vi "Read_spec_No_of_Characters.vi"(0 "Filename":path) -> (1 "character string":string, 2 "Error?":bool)   [LabVIEW 2020]
panel:
  out "error out":errorcluster
  out "Bytes to read":i32
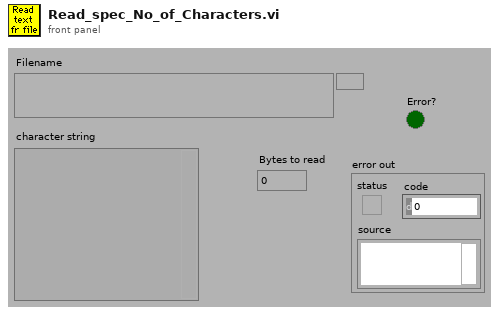
[diagram p1: front panel]
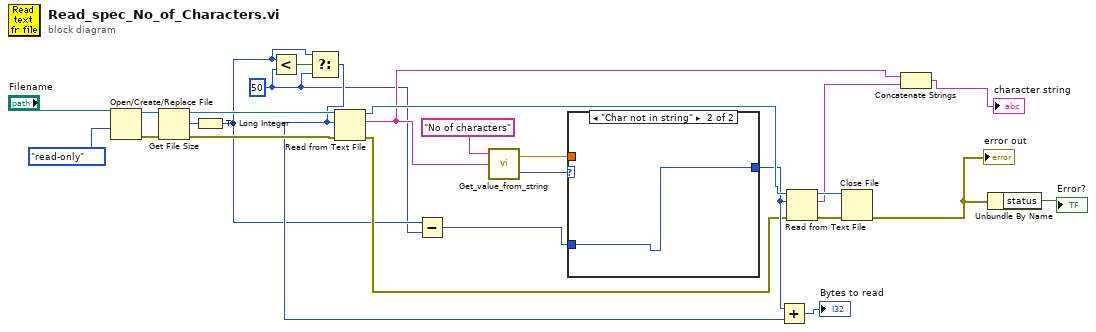
[diagram p0: block diagram]
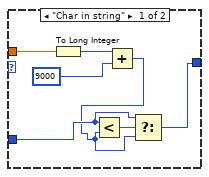
[diagram p2: hidden frame]
diagram:
  w2 = 50 ("number of characters (all:-1)")
  n1 = Open/Create/Replace File(file path (use dialog)="Filename", access (0:read/write)=enum16{"read/write", "read-only", "write-only"}."read-only") -> (refnum out=w17:refnum<file>, error out=w16:errorcluster)  [unwired: 1 in, 4 out]
  n2 = Get File Size(file=w17, error in=w16) -> (refnum out=w15:refnum<file>, size (in bytes)=w12:i64, 0:w14:errorcluster)
  n3 = To Long Integer(number=w12) -> (32bit integer=w3:i32)
  n4 = Less?(x=w3, y=w2) -> (x < y?=w13:bool)
  n5 = Select(t=w3, s=w13, f=w2) -> (s? t:f=w5:i32)
  n6 = Read from Text File(file (use dialog)=w15, count=w5, error in=w14) -> (refnum out=w11:refnum<file>, text=w9:string, error out=w4:errorcluster)  [unwired: 1 in, 1 out]
  n7 = Subtract(x=w3, y=w2) -> (x-y=w1:i32)
  n8 = call "Get_value_from_string.vi"("Input string"=w9, "Variable name"="No of characters") -> ("Status"=w22:enum16{"Char in string", "Char not in string"}, "Value"=w21:dbl)  [unwired: 1 in]
  n9 = case shown="\"Char not in string\"" w22 {
    tunnel: [w27 w34] -> w7
    tunnel: w21 -> [w33 _]
    tunnel: w1 -> [w29 w34]
    frame "Char in string" {
      n10 = To Long Integer(number=w33) -> (32bit integer=w32:i32)
      n11 = Add(x=w32, y=9000) -> (x+y=w28:i32)
      n12 = Less?(x=w29, y=w28) -> (x < y?=w30:bool)
      n13 = Select(t=w29, s=w30, f=w28) -> (s? t:f=w27:i32)
    }
    frame "Char not in string" {
    }
  }
  n14 = Add(x=w7, y=w5) -> (x+y=→"Bytes to read":i32)
  n15 = Read from Text File(file (use dialog)=w11, count=w7, error in=w4) -> (refnum out=w19:refnum<file>, text=w10:string, error out=w20:errorcluster)  [unwired: 1 in, 1 out]
  n16 = Close File(refnum=w19, error in=w20) -> (error out=w24:errorcluster)  [unwired: 1 out]
  "error out" <- w24
  n17 = Concatenate Strings(w9, w10) -> (→"character string":string)
  n18 = Unbundle By Name(w24) -> ("status"=→"Error?":bool)
